vi "_Parse EVM Result.vi"(8 "error in (no error)":errorcluster, 10 "Input String":string, 11 "VISA resource name":refnum<visa-resource-name>) -> (0 "error out":errorcluster, 1 "EVM Results":cluster{"Low Window":dbl, "High Window":dbl}[](array[cluster]) {"High Window" format="%^.3e"; "Low Window" format="%^.3e"}, 2 "Reliability":i32, 3 "VISA resource name out":refnum<visa-resource-name>)   [LabVIEW 2020, in "Rohde&Schwarz CMWXP NR FR1 Measurement.lvlib"]
uses:
  <instrlib>/Rohde&Schwarz CMWXP NR FR1 Measurement/Rohde&Schwarz CMWXP NR FR1 Measurement.lvlib
  <instrlib>/Rohde&Schwarz CMWXP NR FR1 Measurement/Private/rsidr_core.llb/rsidr_core.lvlib
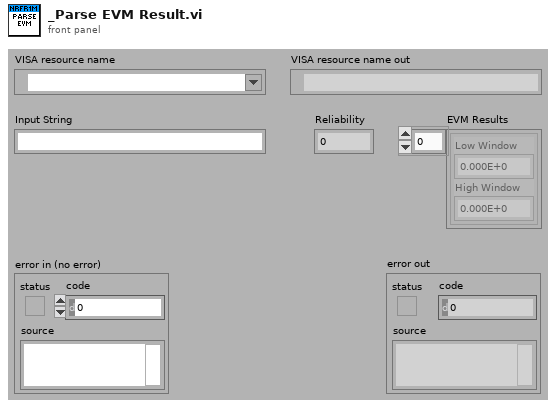
[diagram p1: front panel]
types:
  T1 = cluster{"double value out":dbl, "double value out":dbl}
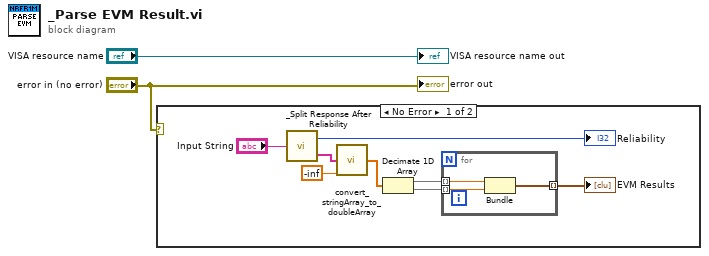
[diagram p0: block diagram]
diagram:
  n1 = case shown="No Error" "error in (no error)" {
    frame No Error {
      n2 = call <instrlib>:"_Split Response After Reliability.vi"("Input String"="Input String") -> ("Response out"=w8:string[], "Reliability out"=→"Reliability":i32)
      n3 = call <instrlib>:"convert_stringArray_to_doubleArray.vi"("default (0)"=-inf, "string array in"=w8) -> ("double array out"=w6:dbl[])  [unwired: 3 in]
      n4 = Decimate 1D Array(w6) -> (w5:dbl[], w4:dbl[])
      n5 = for {
        tunnel: w5 -> [w13] mode=indexing
        tunnel: w4 -> [w12] mode=indexing
        tunnel: [w11] -> w3 mode=indexing
        n6 = Bundle("double value out"=w13, "double value out"=w12) -> (w11:T1)  [unwired: 1 in]
      }
      "EVM Results" <- w3
    }
    frame Error {
    }
  }
  "VISA resource name out" <- "VISA resource name"
  "error out" <- "error in (no error)"
